vi "Host Receiver.vi"() -> ()   [LabVIEW 2010]
doc: "This example demonstrates how to handle communications with multiple servers at once. Each server will ping the host over UDP in order to establish a TCP connection. Once a TCP connection is established, the server and client work in a typical command based fashion. Instead of a single server to communicate with though, the client must handle multiple connections."
uses:
  vi.lib/NI/STM/SubVIs/MetaDataElement.ctl
  vi.lib/NI/STM/Connection Manager/TCP/TCP Connection Method.ctl
  vi.lib/NI/STM/UDP/UDP Read Options.ctl
  vi.lib/NI/STM/Connection Manager/TCP/TCP Connection Properties.ctl
  vi.lib/NI/STM/TCP/TCP Read Options.ctl
  vi.lib/NI/STM/TCP/Get Connection Reference (TCP).vi
  vi.lib/NI/STM/UDP/Set Meta Data (UDP Ref).vi
  vi.lib/NI/STM/TCP/Write Meta Data (TCP Ref).vi
  vi.lib/NI/STM/UDP/Get Connection Reference (UDP).vi
  vi.lib/NI/STM/UDP/Read Message (UDP).vi
  vi.lib/NI/STM/TCP/Write Meta Data (TCP Clst).vi
  vi.lib/NI/STM/TCP/Write Message (TCP).vi
  vi.lib/NI/STM/TCP/Read Message (TCP).vi
  vi.lib/NI/STM/NI STM.lvlib
panel:
  out "error out":errorcluster
  in  "Host Listener Port":u16=5556
  in  "Client Connection Port":u16=5555
  out "Connections":string[](array[string])
  out "Number of \nConnections":i32
  out "Host IP Address":string
  out "New Client IP Address":string
  out "Data from Server 2":dbl[](graph)
  out "Data from Server 1":dbl[](graph)
  in  "stop":bool
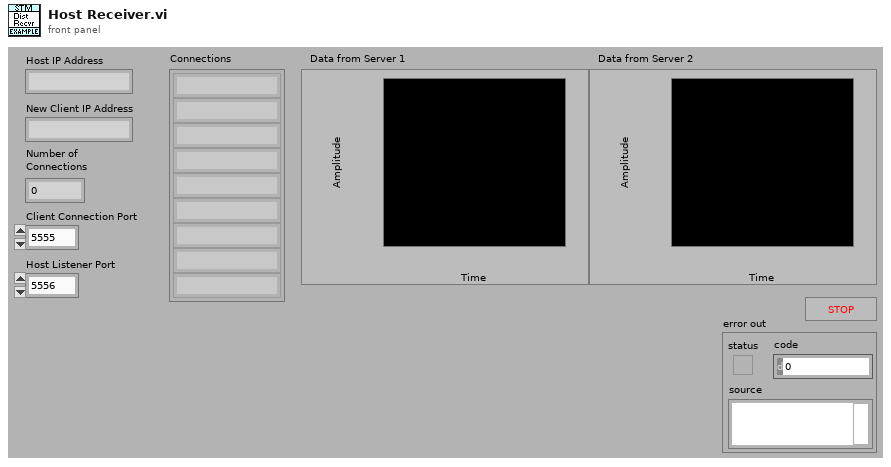
[diagram p1: front panel]
types:
  T1 = typedef "NI STM.lvlib/TCP Connection Method.ctl" = enum16{"Initialize", "Add Connection", "Set Properties", "Get Connection(s)", "Remove Connection", "Remove All Connections", "Get Connection Count"}
  T2 = typedef "NI STM.lvlib/MetaDataElement.ctl" = string
  T3 = typedef "NI STM.lvlib/UDP Connection Info.ctl" = cluster{"connection ID":refnum<k16>, "meta data":T2[]}
  T4 = typedef "NI STM.lvlib/TCP Connection Info.ctl" = cluster{"connection ID":refnum<k5>, "meta data":T2[]}
  T5 = typedef "NI STM.lvlib/TCP Read Options.ctl" = cluster{"ignore timeout error":bool, "timeout ms (1000)":i32}
  T6 = typedef "NI STM.lvlib/TCP Connection Properties.ctl" = cluster{"Name":string, "Address":string, "Custom":string}
  T7 = typedef "NI STM.lvlib/UDP Read Options.ctl" = cluster{"ignore timeout error":bool, "timeout ms (1000)":i32, "max size (548)":i32}
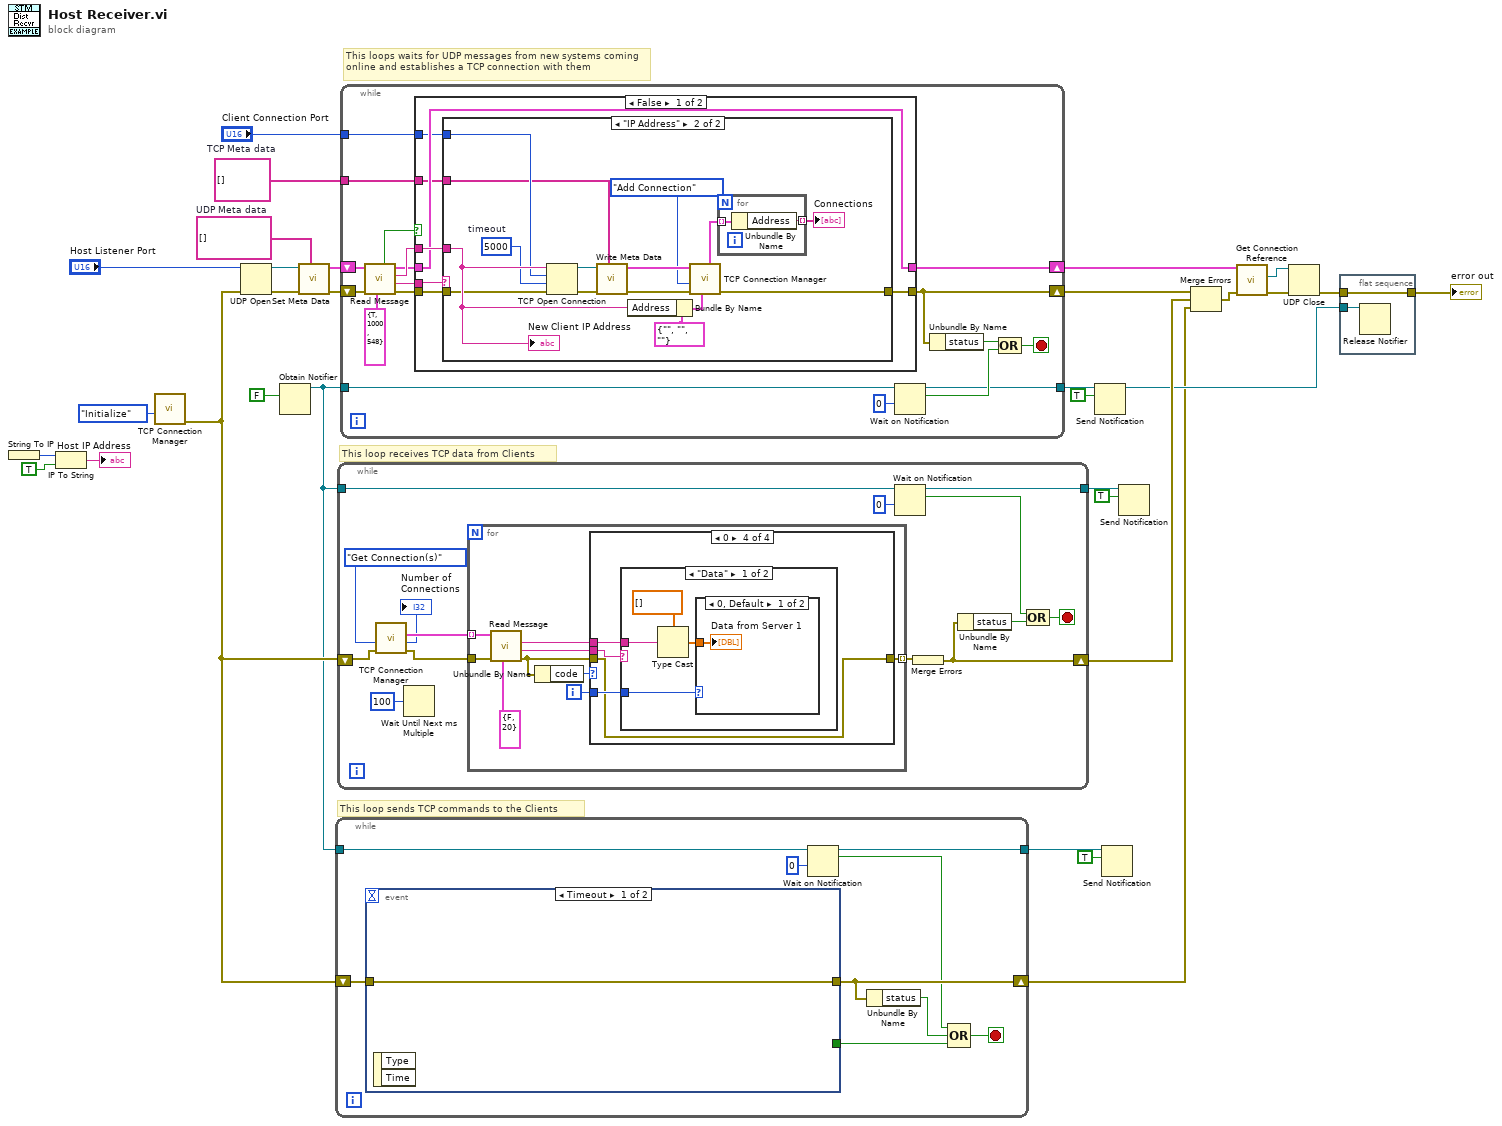
[diagram p0: block diagram]
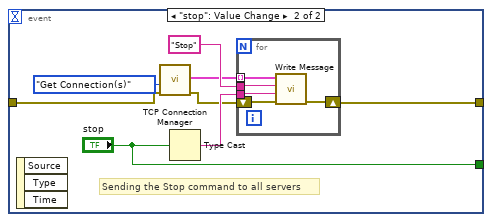
[diagram p4: hidden frame]
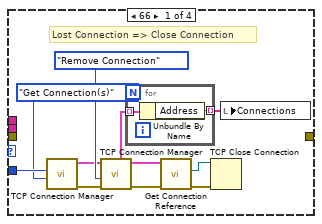
[diagram p5: hidden frame]
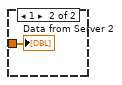
[diagram p8: hidden frame]
diagram:
  w17 = T2[] []  # UDP Meta data
  w30 = T2[] []  # TCP Meta data
  # "This loops waits for UDP messages from new systems coming online and establishes a TCP connection with them"
  # "This loop receives TCP data from Clients"
  # "This loop sends TCP commands to the Clients"
  n1 = String To IP() -> (0:w1:u32)  [unwired: 1 out]
  n2 = IP To String(1:TRUE ("dot notation? (F)"), 2:w1) -> (0:→"Host IP Address":string)
  n3 = call "TCP Connection Manager.vi"("method"=TCP_Connection_Method."Initialize" ("Method")) -> ("error out"=w29:errorcluster)  [unwired: 5 in, 5 out]
  n4 = UDP Open(8:w29, 11:"Host Listener Port") -> (port=w27:refnum<k16>, 0:w28:errorcluster)  [unwired: 3 in, 1 out]
  n5 = Obtain Notifier(notification data type=FALSE) -> (notifier out=w11:refnum<notifier>)  [unwired: 3 in, 2 out]
  n6 = call-poly "Set Meta Data.vi"("meta data"=w17, "error in"=w28, "connection ID"=w27) -> ("error out"=w26:errorcluster, "connection info out"=w25:T3)  [unwired: 7 in]
  n7 = while {
    tunnel: w11 -> [w36]
    tunnel: [w35] -> w9
    shift-right: [w34] -> w5
    shift-left: w29 -> [w40]
    stop <- w38 stop-if-true
    n8 = event shown="[0] Timeout" {
      selector: _ -> [_ _]
      dyn-events: _ -> [_ _]
      timeout: _ -> [_ _]
      tunnel: w40 -> [w41 w44]
      tunnel: [_ "stop"] -> w39
      tunnel: [w41 w42] -> w34
      event Timeout {
        n9 = event-data() -> ()  [unwired: 1 in, 2 out]
      }
      event "stop": Value Change {
        # "Sending the Stop command to all servers"
        n10 = event-data() -> ()  [unwired: 1 in, 3 out]
        n11 = call "TCP Connection Manager.vi"("error in"=w44, "method"=TCP_Connection_Method."Get Connection(s)" ("Method")) -> ("error out"=w43:errorcluster, "all connections"=w46:T4[])  [unwired: 4 in, 4 out]
        n12 = Type Cast(x="stop") -> (*(type *) &x=w48:string)  [unwired: 1 in]
        n13 = for {
          tunnel: "Stop" ("Name") -> [w52]
          tunnel: w48 -> [w51]
          tunnel: w46 -> [w53] mode=indexing
          shift-right: [w50] -> w42
          shift-left: w43 -> [w54]
          n14 = call-poly "Write Message.vi"("error in"=w54, "data"=w51, "name"=w52, "connection info in"=w53) -> ("error out"=w50:errorcluster)  [unwired: 6 in, 1 out]
        }
      }
    }
    n15 = Wait on Notification(notifier=w36, timeout in ms (-1)=0) -> (notifier out=w35:refnum<notifier>, notification=w33:bool)  [unwired: 2 in, 2 out]
    n16 = Unbundle By Name(w34) -> ("status"=w32:bool)
    n17 = Compound Arithmetic op=OR(w33, w32, w39) -> (w38:bool)
  }
  n18 = while {
    tunnel: w11 -> [w61]
    tunnel: [w59] -> w12
    shift-right: [w56] -> w18
    shift-left: w29 -> [w65]
    stop <- w57 stop-if-true
    n19 = call "TCP Connection Manager.vi"("error in"=w65, "method"=TCP_Connection_Method."Get Connection(s)" ("Method")) -> ("error out"=w64:errorcluster, "number of connections"=→"Number of \nConnections":i32, "all connections"=w67:T4[])  [unwired: 4 in, 3 out]
    n20 = Wait Until Next ms Multiple(millisecond multiple=u32 100) -> ()  [unwired: 1 out]
    n21 = for {
      tunnel: w64 -> [w75]
      tunnel: w67 -> [w74] mode=indexing
      tunnel: [w69] -> w62 mode=indexing
      i -> [w73]
      n22 = call-poly "Read Message.vi"("options"=T5 {"ignore timeout error"=FALSE, "timeout ms (1000)"=20} ("Options"), "error in"=w75, "connection info in"=w74) -> ("error out"=w70:errorcluster, "name"=w77:T2, "data string"=w76:string)  [unwired: 3 in, 3 out]
      n23 = Unbundle By Name(w70) -> ("code"=w72:i32)
      n24 = case shown="0" w72 {
        tunnel: w77 -> [_ _ _ w93]
        tunnel: w76 -> [_ _ _ w95]
        tunnel: w73 -> [w81 _ _ w94]
        tunnel: w70 -> [_ _ w91 w92]
        tunnel: [_ _ w91 w92] -> w69
        frame 66 {
          # "Lost Connection => Close Connection"
          n25 = call "TCP Connection Manager.vi"("method"=TCP_Connection_Method."Get Connection(s)" ("Method"), "index"=w81) -> ("error out"=w83:errorcluster, "connection out"=w82:T4)  [unwired: 4 in, 4 out]
          n26 = call "TCP Connection Manager.vi"("error in"=w83, "method"=TCP_Connection_Method."Remove Connection" ("Method"), "connection in"=w82) -> ("error out"=w87:errorcluster, "connection out"=w84:T4, "all properties"=w79:T6[])  [unwired: 3 in, 3 out]
          n27 = for {
            tunnel: w79 -> [w90] mode=indexing
            tunnel: [w89] -> w78 mode=indexing
            n28 = Unbundle By Name(w90) -> ("Address"=w89:string)
          }
          n29 = call-poly "Get Connection Reference.vi"("error in"=w87, "connection info in"=w84) -> ("error out"=w86:errorcluster, "connection ID out"=w85:refnum<k5>)  [unwired: 7 in, 1 out]
          n30 = TCP Close Connection(connection ID=w85, error in (no error)=w86) -> ()  [unwired: 1 in, 2 out]
          n31 = local write "Connections"(w78) -> ()
        }
        frame 56 {
          # "Time out"
        }
        frame Default {
        }
        frame 0 {
          n32 = case shown="\"Data\"" w93 {
            tunnel: w95 -> [w99 _]
            tunnel: w94 -> [w96 _]
            frame "Data" {
              n33 = Type Cast(type=dbl[] [], x=w99) -> (*(type *) &x=w97:dbl[])
              n34 = case shown="0, Default" w96 {
                tunnel: w97 -> [w100 w101]
                frame 0, Default {
                  "Data from Server 1" <- w100
                }
                frame 1 {
                  "Data from Server 2" <- w101
                }
              }
            }
            frame Default {
            }
          }
        }
      }
    }
    n35 = Wait on Notification(notifier=w61, timeout in ms (-1)=0) -> (notifier out=w59:refnum<notifier>, notification=w55:bool)  [unwired: 2 in, 2 out]
    n36 = Merge Errors(w62) -> (w56:errorcluster)
    n37 = Unbundle By Name(w56) -> ("status"=w58:bool)
    n38 = Compound Arithmetic op=OR(w55, w58) -> (w57:bool)
  }
  n39 = while {
    tunnel: w30 -> [w110]
    shift-right: [w112] -> w24
    shift-left: w25 -> [w115]
    shift-right: [w108] -> w20
    shift-left: w26 -> [w119]
    tunnel: "Client Connection Port" -> [w109]
    tunnel: w11 -> [w105]
    tunnel: [w102] -> w15
    stop <- w106 stop-if-true
    n40 = call-poly "Read Message.vi"("options"=T7 {"ignore timeout error"=TRUE, "timeout ms (1000)"=1000, "max size (548)"=548} ("Options"), "error in"=w119, "connection info in"=w115) -> ("error out"=w111:errorcluster, "name"=w116:T2, "data string"=w117:string, "connection info out"=w113:T3, "timed out?"=w118:bool)  [unwired: 3 in, 1 out]
    n41 = case shown="False" w118 {
      tunnel: w117 -> [w126 _]
      tunnel: w116 -> [w125 _]
      tunnel: w113 -> [w124 w146]
      tunnel: [w124 w146] -> w112
      tunnel: w111 -> [w123 w145]
      tunnel: w110 -> [w122 _]
      tunnel: w109 -> [w121 _]
      tunnel: [w120 w145] -> w108
      frame False {
        n42 = case shown="\"IP Address\"" w125 {
          tunnel: w126 -> [_ w138]
          tunnel: w123 -> [w127 w132]
          tunnel: w122 -> [_ w130]
          tunnel: w121 -> [_ w134]
          tunnel: [w127 w131] -> w120
          frame Default {
          }
          frame "IP Address" {
            w133 = 5000  # timeout
            n43 = TCP Open Connection(address=w138, remote port or service name=w134, timeout ms (60000)=w133, error in (no error)=w132) -> (connection ID=w142:refnum<k5>, error out=w141:errorcluster)  [unwired: 1 in]
            n44 = call-poly "Write Meta Data.vi"("meta data"=w130, "error in"=w141, "connection ID"=w142) -> ("error out"=w140:errorcluster, "connection info out"=w139:T4)  [unwired: 7 in]
            n45 = Bundle By Name(cluster=T6 {"Name"="", "Address"="", "Custom"=""} ("Properties In"), "Address"=w138) -> (w135:T6)
            n46 = call "TCP Connection Manager.vi"("properties in"=w135, "error in"=w140, "method"=TCP_Connection_Method."Add Connection" ("Method"), "connection in"=w139) -> ("error out"=w131:errorcluster, "all properties"=w129:T6[])  [unwired: 2 in, 4 out]
            n47 = for {
              tunnel: w129 -> [w144] mode=indexing
              tunnel: [w143] -> w128 mode=indexing
              n48 = Unbundle By Name(w144) -> ("Address"=w143:string)
            }
            "Connections" <- w128
            "New Client IP Address" <- w138
          }
        }
      }
      frame True {
      }
    }
    n49 = Wait on Notification(notifier=w105, timeout in ms (-1)=0) -> (notifier out=w102:refnum<notifier>, notification=w103:bool)  [unwired: 2 in, 2 out]
    n50 = Unbundle By Name(w108) -> ("status"=w107:bool)
    n51 = Compound Arithmetic op=OR(w107, w103) -> (w106:bool)
  }
  n52 = Send Notification(notification=TRUE, notifier=w15) -> (notifier out=w6:refnum<notifier>)  [unwired: 1 in, 1 out]
  n53 = Send Notification(notification=TRUE, notifier=w9) -> ()  [unwired: 1 in, 2 out]
  n54 = Send Notification(notification=TRUE, notifier=w12) -> ()  [unwired: 1 in, 2 out]
  n55 = Merge Errors(w20, w18, w5) -> (w19:errorcluster)
  n56 = call-poly "Get Connection Reference.vi"("error in"=w19, "connection info in"=w24) -> ("error out"=w22:errorcluster, "connection ID"=w23:refnum<k16>)  [unwired: 7 in, 1 out]
  n57 = UDP Close(connection ID=w23, 8:w22) -> (error out=w8:errorcluster)  [unwired: 1 out]
  n58 = flat-sequence {
    tunnel: w8 -> [w148]
    tunnel: [w148] -> w7
    tunnel: w6 -> [w147]
    frame #0 {
      n59 = Release Notifier(notifier=w147) -> ()  [unwired: 2 in, 3 out]
    }
  }
  "error out" <- w7
